vi "user process.vi"(8 "error in":errorcluster, 11 "Parameters to process":T2) -> (0 "error out":errorcluster, 3 "Results from processing":T1)   [LabVIEW 2017, in "Convert Bool to Velocity runtime.lvclass"]
uses:
  Convert Bool to Velocity runtime.lvclass
  parameter user data.ctl
  result user data.ctl
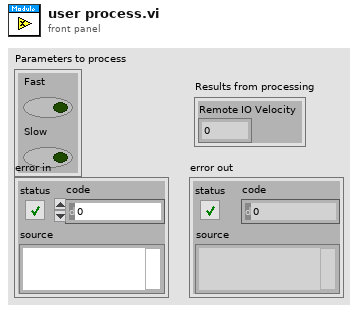
[diagram p1: front panel]
types:
  T1 = typedef "Convert Bool to Velocity runtime.lvclass/result user data.ctl" = cluster{"Remote IO Velocity":dbl}
  T2 = typedef "Convert Bool to Velocity runtime.lvclass/parameter user data.ctl" = cluster{"Fast":bool, "Slow":bool}
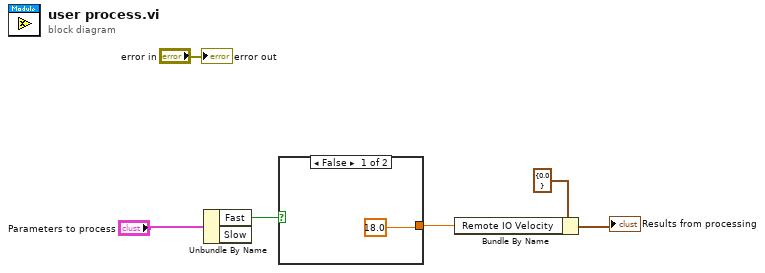
[diagram p0: block diagram]
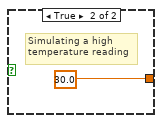
[diagram p2: hidden frame]
diagram:
  n1 = Unbundle By Name("Parameters to process") -> ("Fast"=w2:bool)  [unwired: 1 out]
  n2 = case shown="False" w2 {
    tunnel: [18.0 30.0] -> w1
    frame False {
    }
    frame True {
      # "Simulating a high \ntemperature reading"
    }
  }
  n3 = Bundle By Name(cluster=T1 {"Remote IO Velocity"=0.0} ("Results from processing"), "Remote IO Velocity"=w1) -> (→"Results from processing":T1)
  "error out" <- "error in"
